vi "Get Notifier State.vi"(8 "error in":errorcluster, 11 "Pcal GUI in":refnum<class "Pcal GUI.lvclass">) -> (0 "error out":errorcluster, 2 "Action":u32, 3 "Pcal GUI out":refnum<class "Pcal GUI.lvclass">)   [LabVIEW 2015, in "Pcal GUI.lvclass"]
uses:
  Pcal GUI.lvclass
  Pcal GUI.lvclass/Pcal GUI.ctl
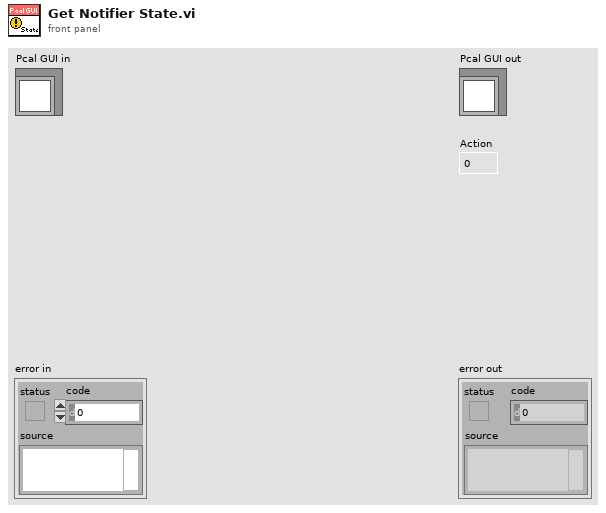
[diagram p1: front panel]
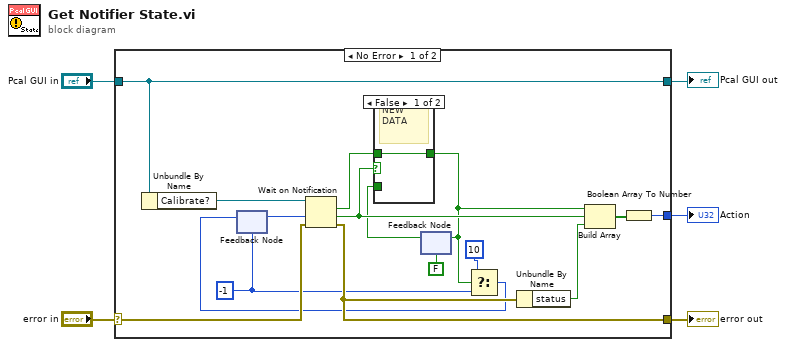
[diagram p0: block diagram]
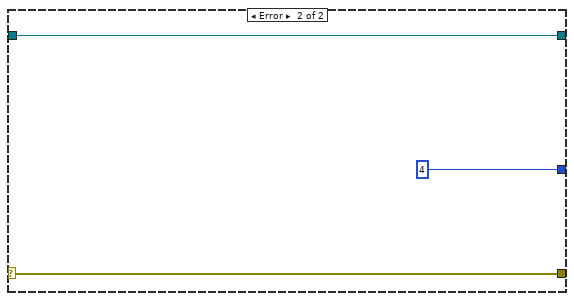
[diagram p3: hidden frame]
diagram:
  n1 = case shown="No Error" "error in" {
    selector: "error in" -> [w14 w26]
    tunnel: [w13 w26] -> w1
    tunnel: [w21 w25] -> w2
    tunnel: "Pcal GUI in" -> [w21 w25]
    tunnel: [w17 u32 4] -> w5
    frame No Error {
      w11 = -1 ("timeout in ms (-1)")
      n2 = Unbundle By Name(w21) -> ("Calibrate?"=w20:refnum<notifier>)
      n3 = feedback #1(w11) -> (w16:i32)
      n4 = Wait on Notification(notifier=w20, timeout in ms (-1)=w16, error in (no error)=w14) -> (notification=w9:bool, timed out?=w10:bool, error out=w13:errorcluster)  [unwired: 1 in, 1 out]
      n5 = feedback #2(FALSE ("timed out?")) -> (w8:bool)
      n6 = case shown="False" w10 {
        tunnel: w9 -> [w22 _]
        tunnel: [w22 w23] -> w6
        tunnel: w8 -> [_ w23]
        frame False {
          # "NEW\nDATA"
        }
        frame True {
          # "TIMED \nOUT"
        }
      }
      n7 = feedback-in #2(w6) -> ()
      n8 = Select(t=10, s=w6, f=w11) -> (s? t:f=w12:i32)
      n9 = feedback-in #1(w12) -> ()
      n10 = Unbundle By Name(w13) -> ("status"=w19:bool)
      n11 = Build Array(w6, w10, w19) -> (w18:bool[])
      n12 = Boolean Array To Number(Boolean array=w18) -> (number=w17:u32)
    }
    frame Error {
    }
  }
  "error out" <- w1
  "Pcal GUI out" <- w2
  "Action" <- w5
